vi "35_Sobel.vi"() -> ()   [LabVIEW 2018]
uses:
  <vilib>/Analysis/2dsp.llb/2D Convolution (DBL).vi
  <vilib>/vision/NI_Vision_Development_Module.lvlib
  <vilib>/Analysis/NI_AALPro.lvlib
panel:
  in  "adj":dbl(slide)=256.0 scale=0.0..500.0
  out "new":T1(plugin-control)
  out "Array":u8[][](array[numeric])
  out "Image 2":T1(plugin-control)
  out "Image Pixels (U8)":u8[][](array[numeric])
  in  "stop":bool
  out "Image":T1(plugin-control)
  # "邊緣檢測 Sobel operator"
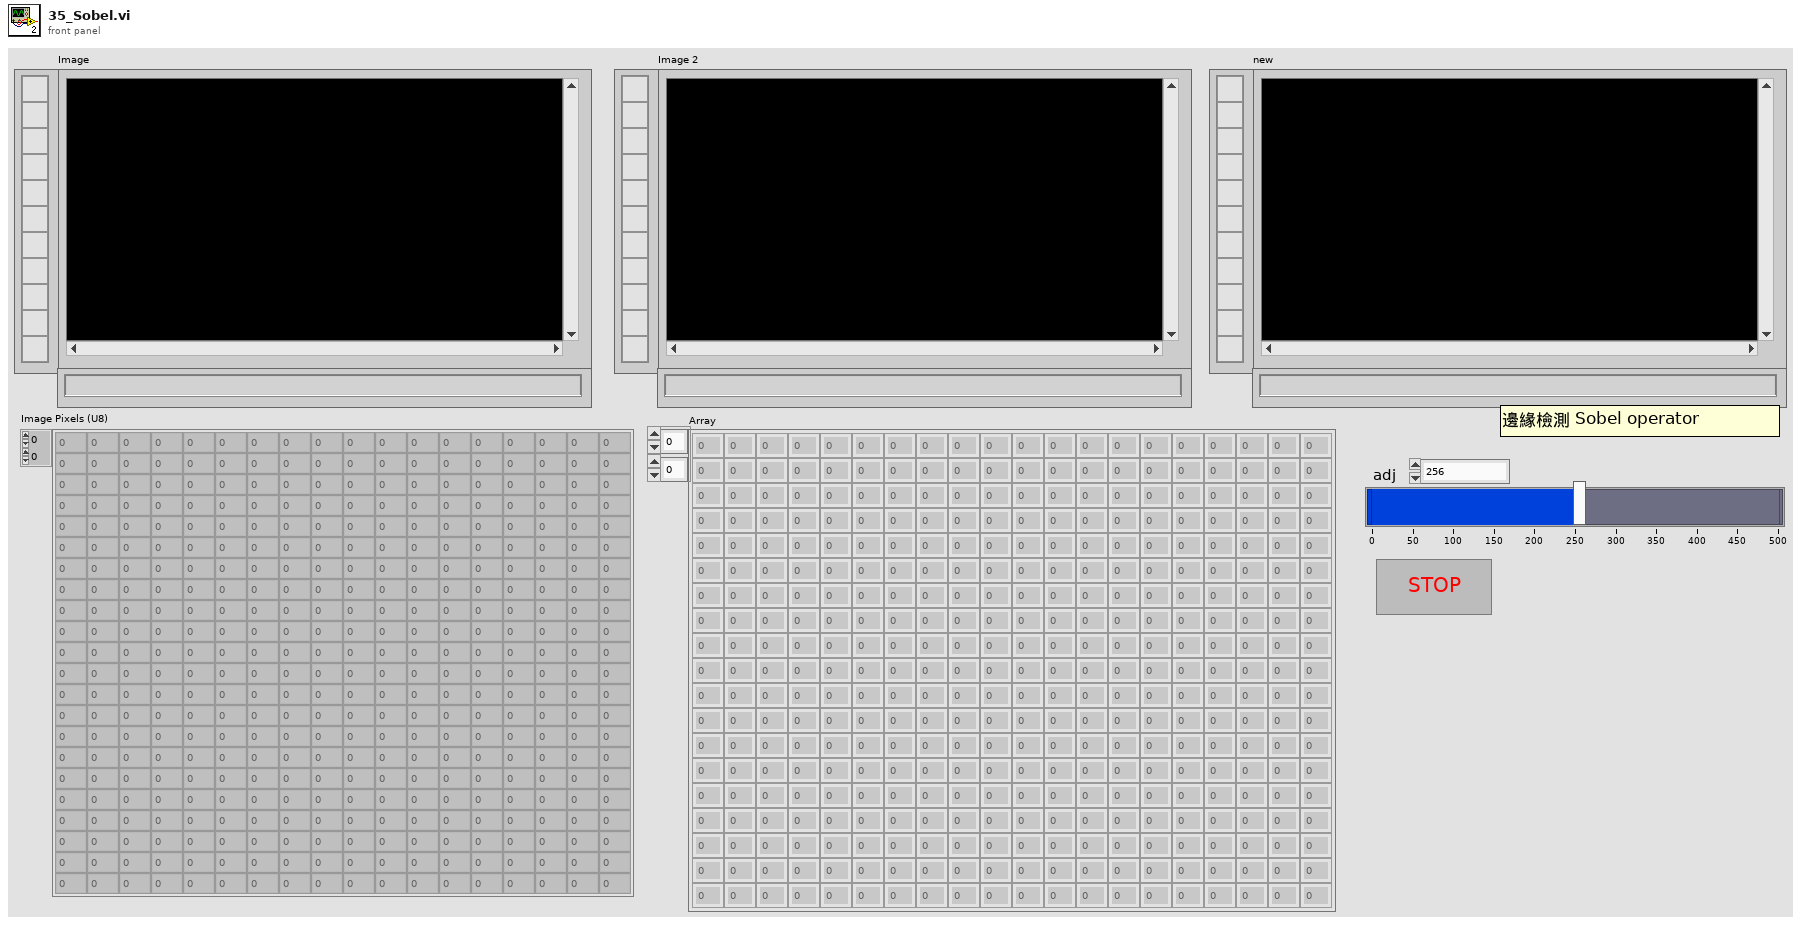
[diagram p1: front panel]
types:
  T1 = typedef "IMAQ Image.ctl" = refnum<image>
  T2 = typedef "Image Type" = u32
  T3 = cluster{"Global Rectangle":i32[], "Contours":cluster{"Contour Type":u32, "ROI Type":u32, "Points":i32[]}[]}
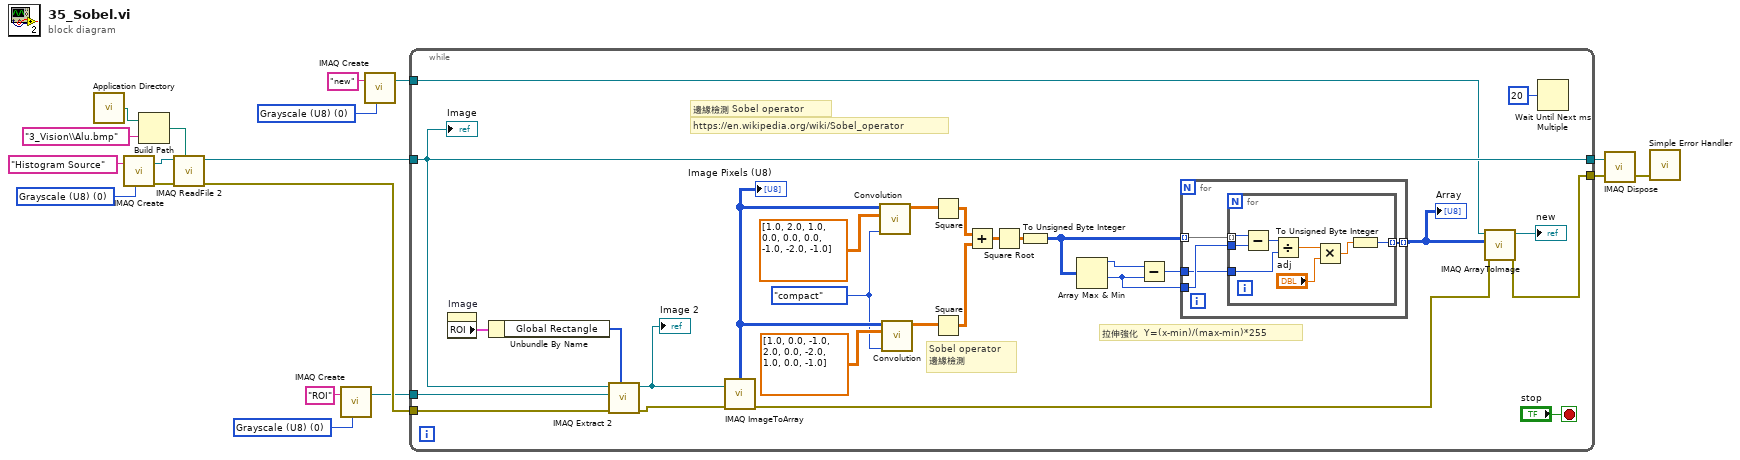
[diagram p0: block diagram]
diagram:
  w2 = T2 0 items=["Grayscale (U8)", "Grayscale (I16)", "Grayscale (SGL)", "Complex (CSG)", "RGB (U32)", "HSL (U32)", "RGB (U64)", "Grayscale (U16)"] ("Image Type")
  w7 = T2 0 items=["Grayscale (U8)", "Grayscale (I16)", "Grayscale (SGL)", "Complex (CSG)", "RGB (U32)", "HSL (U32)", "RGB (U64)", "Grayscale (U16)"] ("Image Type")
  w8 = T2 0 items=["Grayscale (U8)", "Grayscale (I16)", "Grayscale (SGL)", "Complex (CSG)", "RGB (U32)", "HSL (U32)", "RGB (U64)", "Grayscale (U16)"] ("Image Type")
  n1 = call <vilib>:"Application Directory.vi"() -> ("Application Directory"=w10:path)
  n2 = call "IMAQ Create"("Image Name"="Histogram Source", "Image Type"=w8) -> ("New Image"=w18:T1, "error out"=w17:errorcluster)  [unwired: 3 in]
  n3 = Build Path(base path=w10, name or relative path="3_Vision\\Alu.bmp") -> (appended path=w11:path)
  n4 = call "IMAQ ReadFile 2"("File Path"=w11, "error in (no error)"=w17, "Image"=w18) -> ("error out"=w13:errorcluster, "Image Out"=w15:T1)  [unwired: 4 in, 3 out]
  n5 = call "IMAQ Create"("Image Name"="ROI", "Image Type"=w7) -> ("New Image"=w5:T1)  [unwired: 3 in, 1 out]
  n6 = call "IMAQ Create"("Image Name"="new", "Image Type"=w2) -> ("New Image"=w1:T1)  [unwired: 3 in, 1 out]
  n7 = while {
    tunnel: w15 -> [w44]
    tunnel: [w44] -> w14
    tunnel: w13 -> [w41]
    tunnel: w5 -> [w43]
    tunnel: [w35] -> w4
    tunnel: w1 -> [w38]
    stop <- "stop" stop-if-true
    w20 = enum32{"full", "size X", "compact"}."compact" ("output size")
    # "邊緣檢測 Sobel operator"
    # "https://en.wikipedia.org/wiki/Sobel_operator"
    # "拉伸強化  Y=(x-min)/(max-min)*255"
    # "Sobel operator\n邊緣檢測"
    n8 = property on="Image" class="ImageControl"() -> ("ROI"=w45:T3)  [unwired: 2 in, 2 out]
    n9 = Unbundle By Name "Unbundle By Name"(w45) -> ("Global Rectangle"=w42:i32[])
    n10 = call "IMAQ Extract 2"("Optional Rectangle"=w42, "error in (no error)"=w41, "Image Dst"=w43, "Image Src"=w44) -> ("error out"=w39:errorcluster, "Image Dst Out"=w40:T1)  [unwired: 6 in]
    "Image 2" <- w40
    n11 = call "IMAQ ImageToArray"("error in (no error)"=w39, "Image"=w40) -> ("error out"=w36:errorcluster, "Image Pixels (U8)"=w30:u8[][])  [unwired: 2 in, 3 out]
    "Image Pixels (U8)" <- w30
    n12 = call-poly <vilib>:"Convolution.vi"("output size"=w20, "Y"=dbl[][] [[1.0, 2.0, 1.0], [0.0, 0.0, 0.0], [-1.0, -2.0, -1.0]], "X"=w30) -> ("X * Y"=w33:dbl[][])  [unwired: 7 in, 1 out]
    n13 = call-poly <vilib>:"Convolution.vi"("output size"=w20, "Y"=dbl[][] [[1.0, 0.0, -1.0], [2.0, 0.0, -2.0], [1.0, 0.0, -1.0]], "X"=w30) -> ("X * Y"=w31:dbl[][])  [unwired: 7 in, 1 out]
    n14 = Square(x=w33) -> (x^2=w28:dbl[][])
    n15 = Square(x=w31) -> (x^2=w27:dbl[][])
    n16 = Add(x=w28, y=w27) -> (x+y=w29:dbl[][])
    n17 = Square Root(x=w29) -> (sqrt(x)=w26:dbl[][])
    n18 = To Unsigned Byte Integer(number=w26) -> (unsigned 8bit integer=w22:u8[][])
    n19 = Array Max & Min(array=w22) -> (max value=w25:u8, min value=w24:u8)  [unwired: 2 out]
    n20 = Subtract(x=w25, y=w24) -> (x-y=w23:u8)
    n21 = for {
      tunnel: w22 -> [w50] mode=indexing
      tunnel: [w49] -> w21 mode=indexing
      tunnel: w24 -> [w48]
      tunnel: w23 -> [w47]
      n22 = for {
        tunnel: w50 -> [w56] mode=indexing
        tunnel: [w51] -> w49 mode=indexing
        tunnel: w48 -> [w55]
        tunnel: w47 -> [w54]
        n23 = Subtract(x=w56, y=w55) -> (x-y=w58:u8)
        n24 = Divide(x=w58, y=w54) -> (x/y=w57:dbl)
        n25 = Multiply(x=w57, y="adj") -> (x*y=w52:dbl)
        n26 = To Unsigned Byte Integer(number=w52) -> (unsigned 8bit integer=w51:u8)
      }
    }
    "Array" <- w21
    n27 = call "IMAQ ArrayToImage"("error in (no error)"=w36, "Image Pixels (U8)"=w21, "Image"=w38) -> ("error out"=w35:errorcluster, "Image Out"=→"new":T1)  [unwired: 7 in]
    n28 = Wait Until Next ms Multiple(millisecond multiple=u32 20) -> ()  [unwired: 1 out]
    "Image" <- w44
  }
  n29 = call "IMAQ Dispose"("Image"=w14, "error in (no error)"=w4) -> ("error out"=w12:errorcluster)  [unwired: 4 in]
  n30 = call <vilib>:"Simple Error Handler.vi"("error in (no error)"=w12) -> ()  [unwired: 4 in, 5 out]
